vi "testing.vi"() -> ()   [LabVIEW 2009]
panel:
  out "ldr":dbl
  in  "Light,fan/vent":bool[](array[boolean])
  out "shutter, magnet":bool[](array[boolean])
  out "Temp in":dbl(slide) scale=0.0..100.0
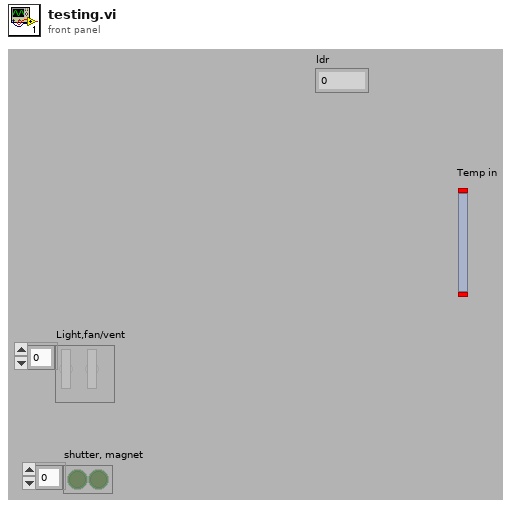
[diagram p1: front panel]
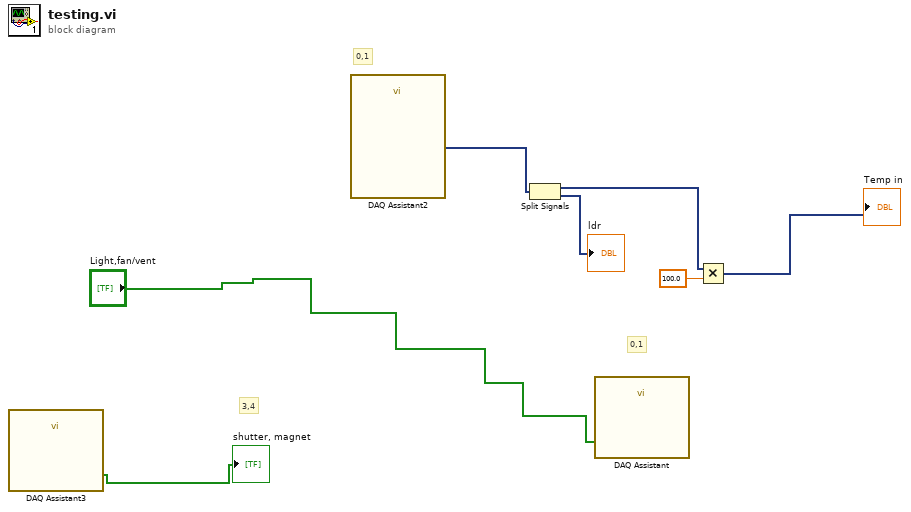
[diagram p0: block diagram]
diagram:
  # "0,1"
  # "0,1"
  # "3,4"
  n1 = call "DAQ Assistant3"() -> ("data"=→"shutter, magnet":bool[])  [unwired: 17 in, 2 out]
  n2 = call "DAQ Assistant2"() -> ("data"=w3:dynamicdata)  [unwired: 17 in, 2 out]
  n3 = Split Signals(w3) -> (w2:dynamicdata, →"ldr":dynamicdata)  [unwired: 2 in]
  n4 = call "DAQ Assistant"("data"="Light,fan/vent") -> ()  [unwired: 17 in, 2 out]
  n5 = Multiply(x=w2, y=100.0) -> (x*y=→"Temp in":dynamicdata)
